vi "Filter Versions.vi"(5 "Older?":bool, 7 "Prerelease?":bool, 11 "WebView2 Updater in":refnum<class "WebView2 Updater.lvclass">) -> (3 "Array":string[](array[string]))   [LabVIEW 2020, in "WebView2 Updater.lvclass"]
uses:
  WebView2 Updater.lvclass
  WebView2 Updater.lvclass/WebView2 Updater.ctl
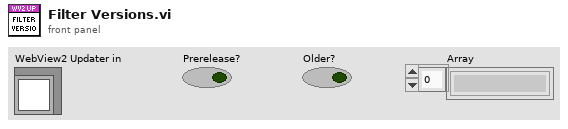
[diagram p1: front panel]
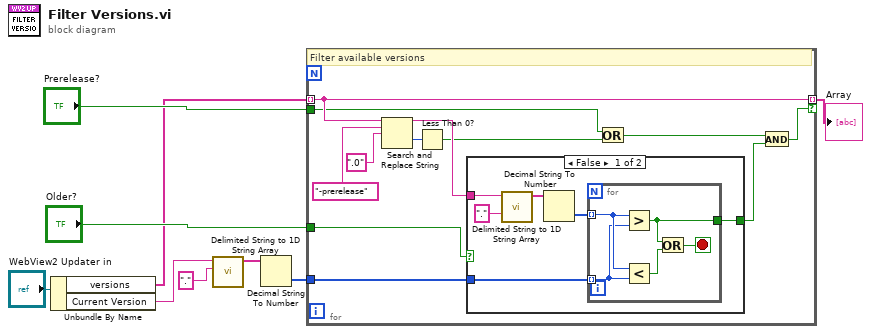
[diagram p0: block diagram]
diagram:
  n1 = Unbundle By Name("WebView2 Updater in") -> ("versions"=w5:string[], "Current Version"=w7:string)
  n2 = call <vilib>:"Delimited String to 1D String Array.vi"("delimiter"=".", "delimited string"=w7) -> ("string array"=w2:string[])  [unwired: 9 in]
  n3 = Decimal String To Number(string=w2) -> (number=w1:i32[])  [unwired: 2 in, 1 out]
  n4 = for {
    tunnel: w5 -> [w17] mode=indexing
    tunnel: w1 -> [w18]
    tunnel: [w17] -> w6 mode=indexing if=w13
    tunnel: "Older?" -> [w11]
    tunnel: "Prerelease?" -> [w10]
    # "Filter available versions"
    n5 = Search and Replace String(input string=w17, search string="-prerelease", replace string=".0" ("replace string (\"\")")) -> (result string=w21:string, offset past replacement=w15:i32)  [unwired: 5 in, 2 out]
    n6 = Less Than 0?(x=w15) -> (x < 0?=w14:bool)
    n7 = case shown="False" w11 {
      selector: w11 -> [_ w33]
      tunnel: w21 -> [w27 _]
      tunnel: w18 -> [w23 _]
      tunnel: [w22 w33] -> w16
      frame False {
        n8 = call <vilib>:"Delimited String to 1D String Array.vi"("delimiter"=".", "delimited string"=w27) -> ("string array"=w25:string[])  [unwired: 9 in]
        n9 = Decimal String To Number(string=w25) -> (number=w24:i32[])  [unwired: 2 in, 1 out]
        n10 = for {
          tunnel: w23 -> [w31] mode=indexing
          tunnel: w24 -> [w32] mode=indexing
          tunnel: [w28] -> w22
          stop <- w29 stop-if-true
          n11 = Greater?(x=w32, y=w31) -> (0:w28:bool)
          n12 = Less?(x=w32, y=w31) -> (x < y?=w30:bool)
          n13 = Or(x=w28, y=w30) -> (x .or. y?=w29:bool)
        }
      }
      frame True {
      }
    }
    n14 = Or(x=w10, y=w14) -> (x .or. y?=w12:bool)
    n15 = And(x=w12, y=w16) -> (x .and. y?=w13:bool)
  }
  "Array" <- w6
